vi "Untitled 1.vi"() -> ()   [LabVIEW 2018]
uses:
  <vilib>/Rock Robotics/Network Tables/NT Write Boolean.vi
  <vilib>/Rock Robotics/Network Tables/NT Write Number.vi
  <vilib>/Rock Robotics/Network Tables/NT Write Numeric Array.vi
panel:
  out "DriveLeftEncoder":dbl
  out "DriveRightEncoder":dbl
  out "Sonar":dbl(graph)
  out "HatchPanelDistance":dbl(graph)
  out "DriveIMU":cluster{"Yaw":dbl, "Pitch":dbl, "Roll":dbl}(graph)
  out "ClimbRearPosition":dbl
  out "ClimbFrontPosition":dbl
  out "Roll":dbl(graph)
  out "Pitch":dbl(graph)
  out "lineIRRearRight":bool
  out "lineIRRearLeft":bool
  out "lineIRFrontRight":bool
  out "lineIRFrontLeft":bool
  out "climbSkidIRRight":bool
  out "climbSkidIRLeft":bool
  out "climbPoweredIRLeft":bool
  out "climbPoweredIRRight":bool
  out "HatchPanelDetect":bool
  out "Yaw":dbl(graph)
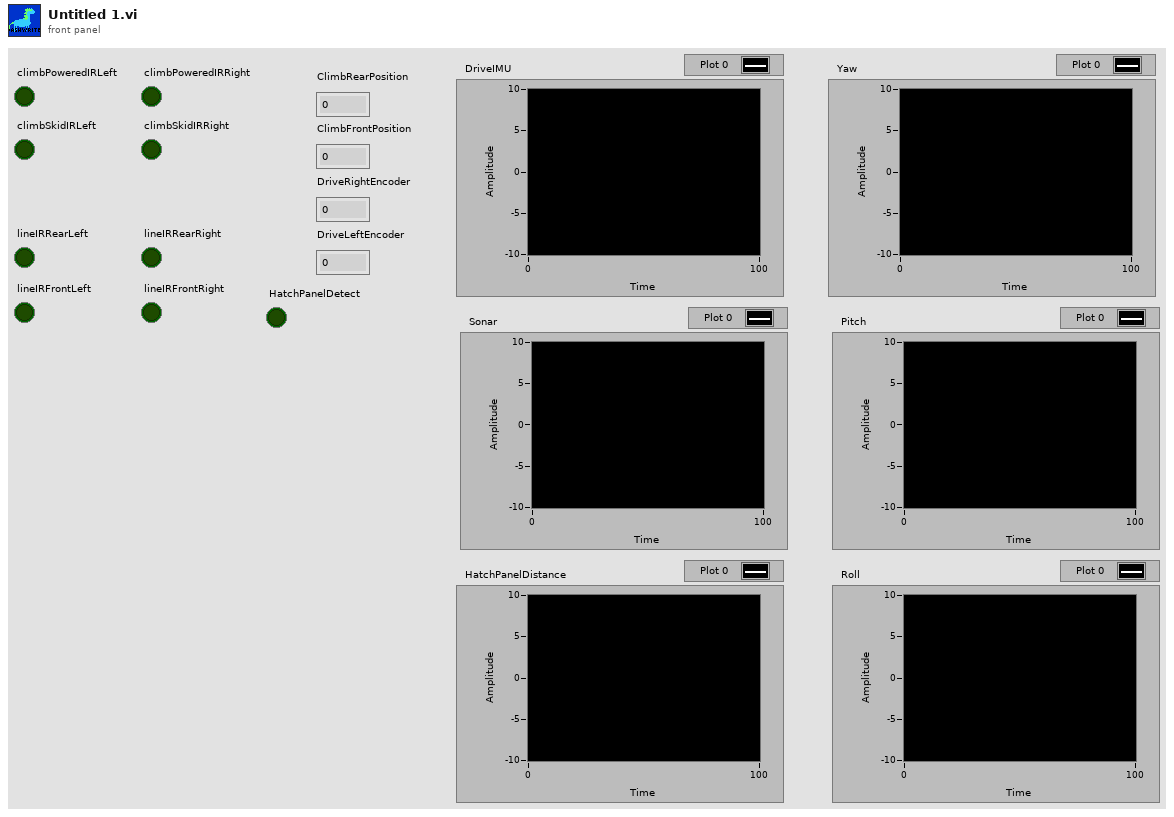
[diagram p1: front panel]
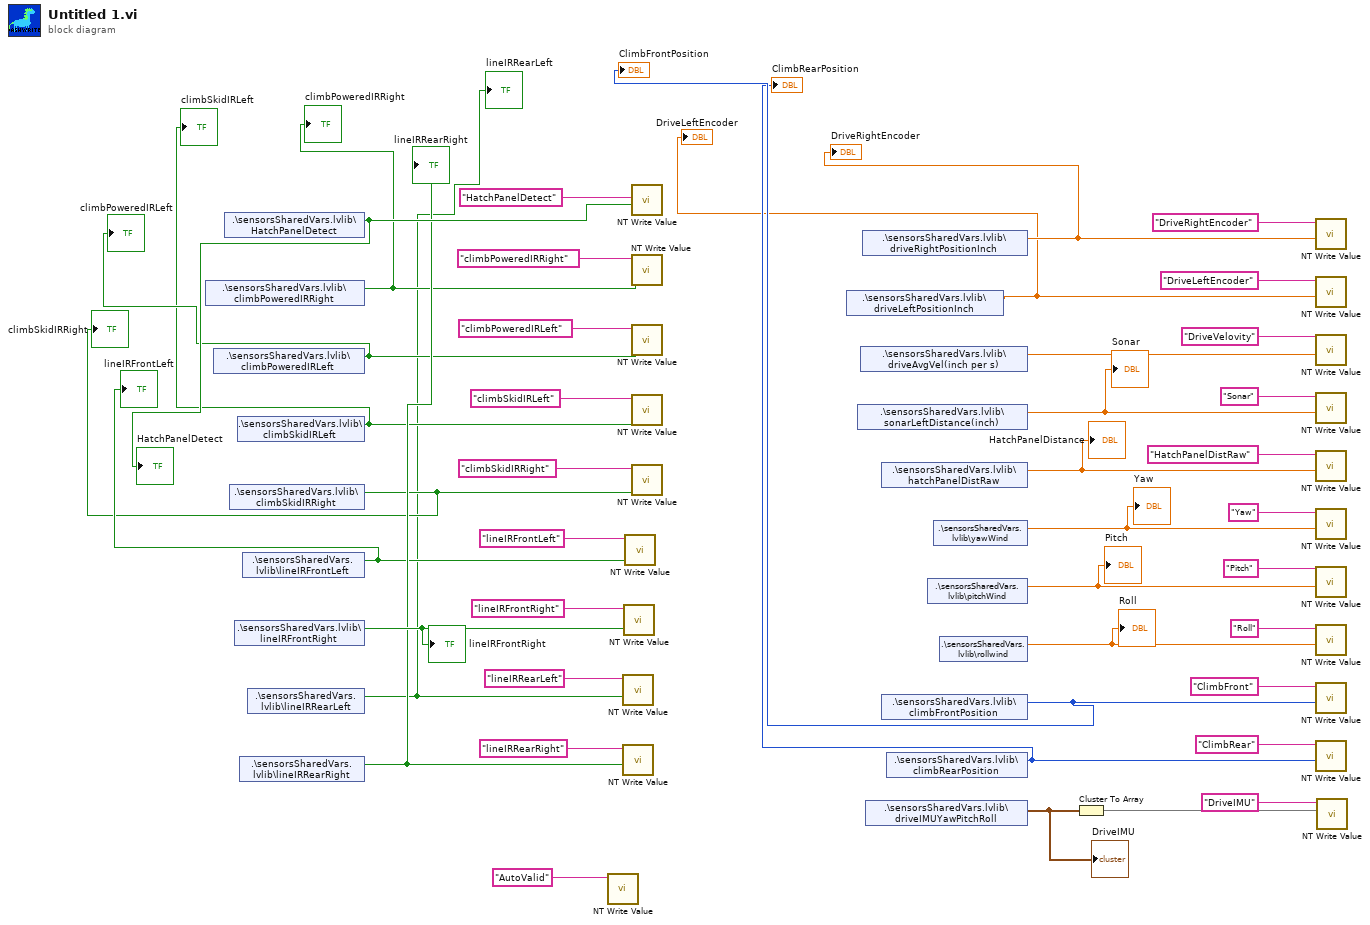
[diagram p0: block diagram]
diagram:
  n1 = shared-variable ".\\sensorsSharedVars.lvlib\\climbPoweredIRRight"() -> (w6:bool)  [unwired: 1 in, 1 out]
  "climbPoweredIRRight" <- w6
  n2 = shared-variable ".\\sensorsSharedVars.lvlib\\climbPoweredIRLeft"() -> (w8:bool)  [unwired: 1 in, 1 out]
  "climbPoweredIRLeft" <- w8
  n3 = shared-variable ".\\sensorsSharedVars.lvlib\\HatchPanelDetect"() -> (w12:bool)  [unwired: 1 in, 1 out]
  "HatchPanelDetect" <- w12
  n4 = shared-variable ".\\sensorsSharedVars.lvlib\\climbSkidIRRight"() -> (w9:bool)  [unwired: 1 in, 1 out]
  "climbSkidIRRight" <- w9
  n5 = shared-variable ".\\sensorsSharedVars.lvlib\\lineIRFrontRight"() -> (w13:bool)  [unwired: 1 in, 1 out]
  "lineIRFrontRight" <- w13
  n6 = shared-variable ".\\sensorsSharedVars.lvlib\\climbSkidIRLeft"() -> (w7:bool)  [unwired: 1 in, 1 out]
  "climbSkidIRLeft" <- w7
  n7 = shared-variable ".\\sensorsSharedVars.lvlib\\lineIRRearRight"() -> (w11:bool)  [unwired: 1 in, 1 out]
  "lineIRRearRight" <- w11
  n8 = shared-variable ".\\sensorsSharedVars.lvlib\\lineIRFrontLeft"() -> (w10:bool)  [unwired: 1 in, 1 out]
  "lineIRFrontLeft" <- w10
  n9 = shared-variable ".\\sensorsSharedVars.lvlib\\lineIRRearLeft"() -> (w5:bool)  [unwired: 1 in, 1 out]
  "lineIRRearLeft" <- w5
  n10 = call-poly <vilib>:"NT Write Value.vi"("Name"="AutoValid") -> ()  [unwired: 10 in, 1 out]
  n11 = call-poly <vilib>:"NT Write Value.vi"("Boolean"=w5, "Name"="lineIRRearLeft") -> ()  [unwired: 9 in, 1 out]
  n12 = call-poly <vilib>:"NT Write Value.vi"("Boolean"=w11, "Name"="lineIRRearRight") -> ()  [unwired: 9 in, 1 out]
  n13 = call-poly <vilib>:"NT Write Value.vi"("Boolean"=w13, "Name"="lineIRFrontRight") -> ()  [unwired: 9 in, 1 out]
  n14 = call-poly <vilib>:"NT Write Value.vi"("Boolean"=w10, "Name"="lineIRFrontLeft") -> ()  [unwired: 9 in, 1 out]
  n15 = call-poly <vilib>:"NT Write Value.vi"("Boolean"=w12, "Name"="HatchPanelDetect") -> ()  [unwired: 9 in, 1 out]
  n16 = call-poly <vilib>:"NT Write Value.vi"("Boolean"=w6, "Name"="climbPoweredIRRight") -> ()  [unwired: 9 in, 1 out]
  n17 = call-poly <vilib>:"NT Write Value.vi"("Boolean"=w8, "Name"="climbPoweredIRLeft") -> ()  [unwired: 9 in, 1 out]
  n18 = call-poly <vilib>:"NT Write Value.vi"("Boolean"=w7, "Name"="climbSkidIRLeft") -> ()  [unwired: 9 in, 1 out]
  n19 = call-poly <vilib>:"NT Write Value.vi"("Boolean"=w9, "Name"="climbSkidIRRight") -> ()  [unwired: 9 in, 1 out]
  n20 = shared-variable ".\\sensorsSharedVars.lvlib\\driveLeftPositionInch"() -> (w1:dbl)  [unwired: 1 in, 1 out]
  "DriveLeftEncoder" <- w1
  n21 = shared-variable ".\\sensorsSharedVars.lvlib\\sonarLeftDistance(inch)"() -> (w14:dbl)  [unwired: 1 in, 1 out]
  "Sonar" <- w14
  n22 = shared-variable ".\\sensorsSharedVars.lvlib\\driveAvgVel(inch per s)"() -> (w40:dbl)  [unwired: 1 in, 1 out]
  n23 = shared-variable ".\\sensorsSharedVars.lvlib\\driveRightPositionInch"() -> (w3:dbl)  [unwired: 1 in, 1 out]
  "DriveRightEncoder" <- w3
  n24 = shared-variable ".\\sensorsSharedVars.lvlib\\driveIMUYawPitchRoll"() -> (w19:cluster{"Yaw":dbl, "Pitch":dbl, "Roll":dbl})  [unwired: 1 in, 1 out]
  "DriveIMU" <- w19
  n25 = shared-variable ".\\sensorsSharedVars.lvlib\\hatchPanelDistRaw"() -> (w16:dbl)  [unwired: 1 in, 1 out]
  "HatchPanelDistance" <- w16
  n26 = shared-variable ".\\sensorsSharedVars.lvlib\\climbFrontPosition"() -> (w4:i32)  [unwired: 1 in, 1 out]
  "ClimbFrontPosition" <- w4
  n27 = shared-variable ".\\sensorsSharedVars.lvlib\\climbRearPosition"() -> (w2:i32)  [unwired: 1 in, 1 out]
  "ClimbRearPosition" <- w2
  n28 = shared-variable ".\\sensorsSharedVars.lvlib\\pitchWind"() -> (w17:dbl)  [unwired: 1 in, 1 out]
  "Pitch" <- w17
  n29 = shared-variable ".\\sensorsSharedVars.lvlib\\yawWind"() -> (w15:dbl)  [unwired: 1 in, 1 out]
  "Yaw" <- w15
  n30 = shared-variable ".\\sensorsSharedVars.lvlib\\rollwind"() -> (w18:dbl)  [unwired: 1 in, 1 out]
  "Roll" <- w18
  n31 = Cluster To Array(cluster=w19) -> (array=w41:dbl[])
  n32 = call-poly <vilib>:"NT Write Value.vi"("Numeric"=w3, "Name"="DriveRightEncoder") -> ()  [unwired: 9 in, 1 out]
  n33 = call-poly <vilib>:"NT Write Value.vi"("Numeric"=w1, "Name"="DriveLeftEncoder") -> ()  [unwired: 9 in, 1 out]
  n34 = call-poly <vilib>:"NT Write Value.vi"("Numeric"=w40, "Name"="DriveVelovity") -> ()  [unwired: 9 in, 1 out]
  n35 = call-poly <vilib>:"NT Write Value.vi"("Numeric"=w14, "Name"="Sonar") -> ()  [unwired: 9 in, 1 out]
  n36 = call-poly <vilib>:"NT Write Value.vi"("Numeric"=w16, "Name"="HatchPanelDistRaw") -> ()  [unwired: 9 in, 1 out]
  n37 = call-poly <vilib>:"NT Write Value.vi"("Numeric"=w15, "Name"="Yaw") -> ()  [unwired: 9 in, 1 out]
  n38 = call-poly <vilib>:"NT Write Value.vi"("Numeric"=w17, "Name"="Pitch") -> ()  [unwired: 9 in, 1 out]
  n39 = call-poly <vilib>:"NT Write Value.vi"("Numeric"=w18, "Name"="Roll") -> ()  [unwired: 9 in, 1 out]
  n40 = call-poly <vilib>:"NT Write Value.vi"("Numeric"=w4, "Name"="ClimbFront") -> ()  [unwired: 9 in, 1 out]
  n41 = call-poly <vilib>:"NT Write Value.vi"("Numeric"=w2, "Name"="ClimbRear") -> ()  [unwired: 9 in, 1 out]
  n42 = call-poly <vilib>:"NT Write Value.vi"("Numeric Array"=w41, "Name"="DriveIMU") -> ()  [unwired: 9 in, 1 out]
